vi "VPI Set PWM Period.vi"(7 "pFrequency":u32, 9 "ChannelMask":u8, 10 "DevIndex":i32, 11 "DevType":i32) -> (3 "function return":i32, 5 "pFrequency out":u32)   [LabVIEW 2010, in "ControlPWM.lvlib"]
doc: "int WINAPI VPI_SetPWMPeriod(int DevType, int DevIndex, unsigned char ChannelMask,unsigned int *pFrequency);"
uses:
  ControlPWM.lvlib
  ControlPWM/Ginkgo_Driver.dll
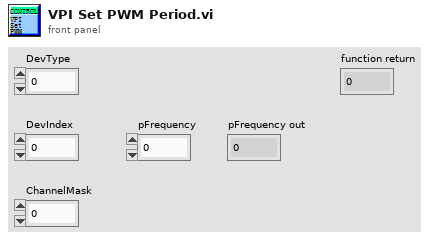
[diagram p1: front panel]
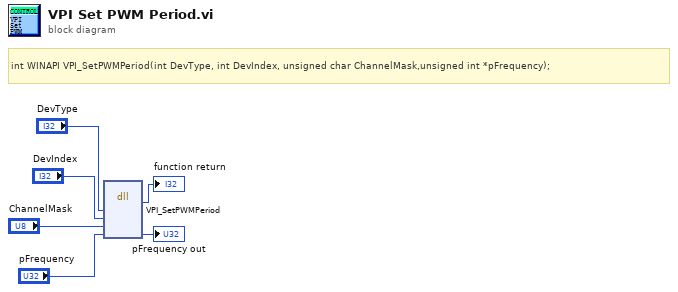
[diagram p0: block diagram]
diagram:
  # "int\tWINAPI VPI_SetPWMPeriod(int DevType, int DevIndex, unsigned char ChannelMask,unsigned int *pFrequency);"
  n1 = dll-call lib="E:/Project/vt_ginkgo/truck/Ginkgo Driver/vs2010/Ginkgo_USB-I2C&SPI&CAN_API_v2.0.3.3/lib/labview_32bit/ControlPWM/Ginkgo_Driver.*" fn="VPI_SetPWMPeriod"("DevType"="DevType", "DevIndex"="DevIndex", "ChannelMask"="ChannelMask", "pFrequency"="pFrequency") -> (→"function return":i32, "pFrequency"=→"pFrequency out":u32)  [unwired: 6 in, 2 out]
